vi "Update Barrel.vi"(8 "error in (no error)":errorcluster, 11 "PL Model Data in":T1={"Position"=0.0, "Settings"={"Length [m]"=20.0, "Dose Zone Start"=8.0, "Dose Zone  End"=12.0, "Barrel Volume [l]"=100.0, "Dosing level [l]"=90.0}, "Pump State"=FALSE, "Fluid Flow"=0.0, "Inpute Zone"=FALSE, "Dosing Zone"=FALSE, "Output Zone"=FALSE, "UI Refs"={"DOSING"=refnum, "INPUT"=refnum, "OUTPUT"=refnum, "Pump"=refnum, "Fluid Level [l]"=refnum, "Flow [l/s]"=refnum, "Production line"=refnum, "SPILL"=refnum, "LOW LEVEL"=refnum, "Barrel Number"=refnum}, "Fluid Level"=0.0, "Barrel Number"=0, "Spill Alarm"=FALSE, "Level Alarm"=FALSE, "millisecond timer value"=0, "Start simulation"=FALSE}) -> (0 "error out":errorcluster, 3 "PL Model Data out":T1={"Position"=0.0, "Settings"={"Length [m]"=20.0, "Dose Zone Start"=8.0, "Dose Zone  End"=12.0, "Barrel Volume [l]"=100.0, "Dosing level [l]"=90.0}, "Pump State"=FALSE, "Fluid Flow"=0.0, "Inpute Zone"=FALSE, "Dosing Zone"=FALSE, "Output Zone"=FALSE, "UI Refs"={"DOSING"=refnum, "INPUT"=refnum, "OUTPUT"=refnum, "Pump"=refnum, "Fluid Level [l]"=refnum, "Flow [l/s]"=refnum, "Production line"=refnum, "SPILL"=refnum, "LOW LEVEL"=refnum, "Barrel Number"=refnum}, "Fluid Level"=0.0, "Barrel Number"=0, "Spill Alarm"=FALSE, "Level Alarm"=FALSE, "millisecond timer value"=0, "Start simulation"=FALSE})   [LabVIEW 2014, in "Model.lvlib"]
uses:
  Model.lvlib
  TypeDefs/PL Settings.ctl
  TypeDefs/PL UI Refs.ctl
  TypeDefs/Model Data.ctl
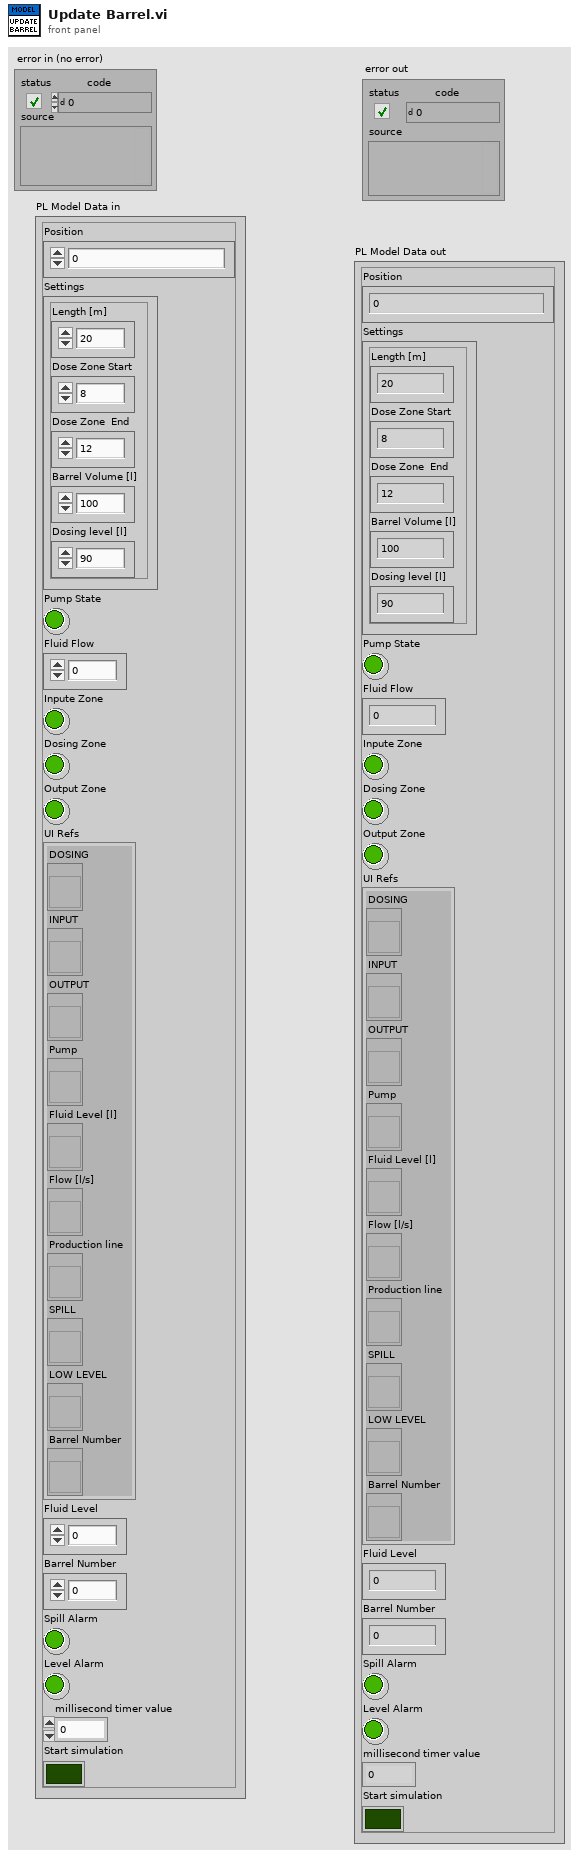
[diagram p1: front panel]
types:
  T1 = typedef "Model.lvlib/Model Data.ctl" = cluster{"Position":dbl, "Settings":T2, "Pump State":bool, "Fluid Flow":dbl, "Inpute Zone":bool, "Dosing Zone":bool, "Output Zone":bool, "UI Refs":T3, "Fluid Level":dbl, "Barrel Number":i32, "Spill Alarm":bool, "Level Alarm":bool, "millisecond timer value":u32, "Start simulation":bool}
  T2 = typedef "Model.lvlib/PL Settings.ctl" = cluster{"Length [m]":dbl, "Dose Zone Start":dbl, "Dose Zone  End":dbl, "Barrel Volume [l]":dbl, "Dosing level [l]":dbl}
  T3 = typedef "Model.lvlib/PL UI Refs.ctl" = cluster{"DOSING":refnum<vi>, "INPUT":refnum<vi>, "OUTPUT":refnum<vi>, "Pump":refnum<vi>, "Fluid Level [l]":refnum<vi>, "Flow [l/s]":refnum<vi>, "Production line":refnum<vi>, "SPILL":refnum<vi>, "LOW LEVEL":refnum<vi>, "Barrel Number":refnum<vi>}
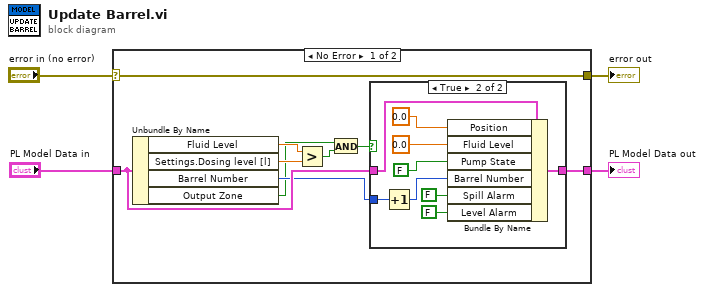
[diagram p0: block diagram]
diagram:
  n1 = case shown="No Error" "error in (no error)" {
    selector: "error in (no error)" -> [w8 w24]
    tunnel: "PL Model Data in" -> [w11 w25]
    tunnel: [w10 w25] -> w3
    tunnel: [w8 w24] -> w1
    frame No Error {
      n2 = Unbundle By Name(w11) -> ("Fluid Level"=w13:dbl, "Settings.Dosing level [l]"=w12:dbl, "Barrel Number"=w9:i32, "Output Zone"=w7:bool)
      n3 = Greater?(x=w13, y=w12) -> (0:w6:bool)
      n4 = And(x=w7, y=w6) -> (x .and. y?=w5:bool)
      n5 = case shown="True" w5 {
        tunnel: w11 -> [w14 w23]
        tunnel: [w14 w22] -> w10
        tunnel: w9 -> [_ w21]
        frame False {
        }
        frame True {
          n6 = Increment(x=w21) -> (x+1=w17:i32)
          n7 = Bundle By Name(cluster=w23, "Position"=0.0, "Fluid Level"=0.0, "Pump State"=FALSE, "Barrel Number"=w17, "Spill Alarm"=FALSE, "Level Alarm"=FALSE) -> (w22:T1)
        }
      }
    }
    frame Error {
    }
  }
  "PL Model Data out" <- w3
  "error out" <- w1
